vi "Clean3DArray.vi"(10 "3D Array":T1[](array[typedef])) -> (2 "Array3DClean":T1[](array[typedef]))   [LabVIEW 2020]
uses:
  _Controls/3DData.ctl
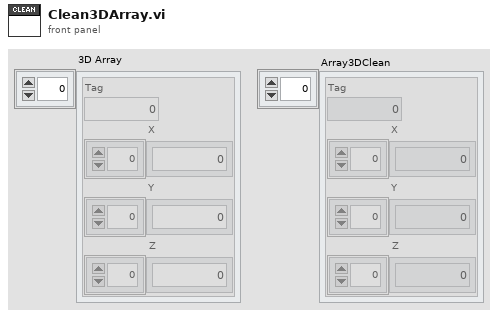
[diagram p1: front panel]
types:
  T1 = typedef "3DData.ctl" = cluster{"Tag":i32, "X":dbl[], "Y":dbl[], "Z":dbl[]}
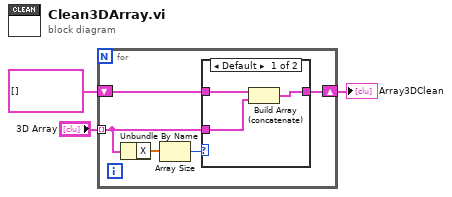
[diagram p0: block diagram]
diagram:
  n1 = for {
    tunnel: "3D Array" -> [w4] mode=indexing
    shift-right: [w5] -> w1
    shift-left: T1[] [] -> [w6]
    n2 = Unbundle By Name(w4) -> ("X"=w8:dbl[])
    n3 = Array Size(array=w8) -> (size(s)=w7:i32)
    n4 = case shown="Default" w7 {
      tunnel: w6 -> [w11 w12]
      tunnel: [w9 w12] -> w5
      tunnel: w4 -> [w10 _]
      frame Default {
        n5 = Build Array (concatenate)(w11, w10) -> (w9:T1[])
      }
      frame 0 {
      }
    }
  }
  "Array3DClean" <- w1
